vi "SetSingleIM.vi"(6 "Legacy (f)?":bool, 8 "error in (no error)":errorcluster, 10 "SingleIM?":bool) -> (0 "error out":errorcluster)   [LabVIEW 2011]
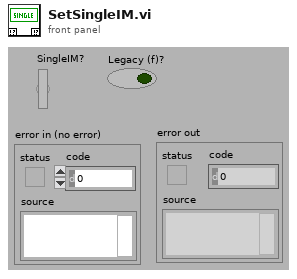
[diagram p1: front panel]
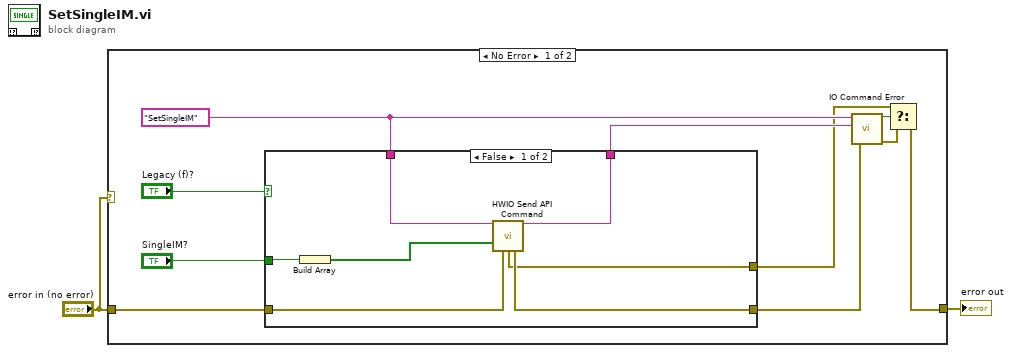
[diagram p0: block diagram]
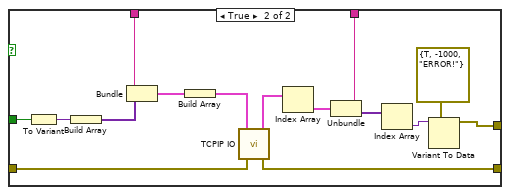
[diagram p2: hidden frame]
diagram:
  n1 = case shown="No Error" "error in (no error)" {
    tunnel: "error in (no error)" -> [w11 w35]
    tunnel: [w5 w35] -> w2
    frame No Error {
      w10 = "SetSingleIM"
      n2 = case shown="False" "Legacy (f)?" {
        tunnel: "SingleIM?" -> [w15 w34]
        tunnel: w11 -> [w17 w31]
        tunnel: w10 -> [w19 w29]
        tunnel: [w16 w28] -> w9
        tunnel: [w18 w24] -> w8
        tunnel: [w13 w20] -> w4
        frame False {
          n3 = Build Array(w15) -> (w14:bool[])
          n4 = call "HWIO Send API Command.vi"("Action"=w19, "Boolean"=w14, "error in (no error)"=w17) -> ("Action out"=w18:string, "HWError"=w13:errorcluster, "error out"=w16:errorcluster)  [unwired: 5 in, 5 out]
        }
        frame True {
          n5 = To Variant(anything=w34) -> (Variant=w33:variant)
          n6 = Build Array(w33) -> (w32:variant[])
          n7 = Bundle(w29, w32) -> (w30:cluster{string, variant[]})  [unwired: 1 out]
          n8 = Build Array(w30) -> (w27:cluster{string, variant[]}[])
          n9 = call "TCPIP IO.vi"("error in (no error)"=w31, "Commands"=w27) -> ("error out"=w28:errorcluster, "Responses"=w25:cluster{string, variant[]}[])  [unwired: 1 in, 3 out]
          n10 = Index Array(array=w25) -> (element=w26:cluster{string, variant[]})  [unwired: 1 in]
          n11 = Unbundle(w26) -> (w24:string, w21:variant[])
          n12 = Index Array(array=w21) -> (element=w23:variant)  [unwired: 1 in]
          n13 = Variant To Data(type=errorcluster {"status"=TRUE, "code"=-1000, "source"="ERROR!"} ("error out"), Variant=w23) -> (data=w20:errorcluster)  [unwired: 1 in, 1 out]
        }
      }
      n14 = call "IO Command Error.vi"("error in (no error)"=w9, "Command Returned (\"\")"=w8, "Command Sent (\"\")"=w10) -> ("error out"=w6:errorcluster, "HW ERR?"=w7:bool)  [unwired: 3 out]
      n15 = Select(t=w4, s=w7, f=w6) -> (s? t:f=w5:errorcluster)
    }
    frame Error {
    }
  }
  "error out" <- w2
